vi "Show Log Viewer.vi"   [LabVIEW 2015]
types:
  T1 = enum32{"Bad", "Idle", "Run top level", "Running"}
  T2 = enum32{"Invalid", "Standard", "Closed", "Hidden", "Minimized", "Maximized"}
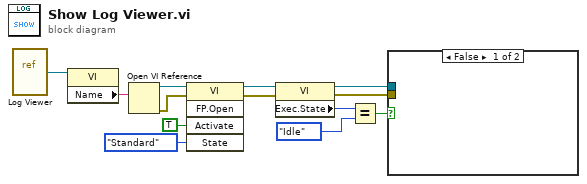
[diagram p0: block diagram]
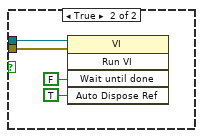
[diagram p2: hidden frame]
diagram:
  n1 = vi-ref "Log Viewer.vi"() -> (w13:refnum<vi>)
  n2 = property class="VI"(reference=w13) -> ("Name"=w12:string)  [unwired: 1 in, 2 out]
  n3 = Open VI Reference(vi path=w12) -> (vi reference=w11:refnum<vi>, error out=w10:errorcluster)  [unwired: 5 in]
  n4 = invoke class="VI" method="FP.Open"(reference=w11, error in=w10, "Activate"=TRUE ("Activate?"), "State"=T2."Standard") -> (reference out=w7:refnum<vi>, error out=w6:errorcluster)  [unwired: 1 in, 3 out]
  n5 = property class="VI"(reference=w7, error in=w6) -> (reference out=w3:refnum<vi>, error out=w2:errorcluster, "Exec.State"=w5:T1)
  n6 = Equal?(x=w5, y=T1."Idle") -> (x = y?=w1:bool)
  n7 = case shown="False" w1 {
    tunnel: w3 -> [_ w15]
    tunnel: w2 -> [_ w14]
    frame False {
    }
    frame True {
      n8 = invoke class="VI" method="Run VI"(reference=w15, error in=w14, "Wait until done"=FALSE ("Wait Until Done"), "Auto Dispose Ref"=TRUE ("Auto Dispose Reference")) -> ()  [unwired: 1 in, 5 out]
    }
  }
